vi "tsdiag_can_transfer_data.vi"(6 "AReqCase":i32, 7 "ADataSize":i32, 8 "error in (no error)":errorcluster, 9 "ASourceData":u8[](array[numeric]), 10 "ADiagModuleIndex":i32, 11 "路径输入":path) -> (0 "error out":errorcluster, 1 "Succes？":bool, 2 "return":i32, 3 "路径输出":path)   [LabVIEW 2014]
doc: "36服务，请求传输数据。"
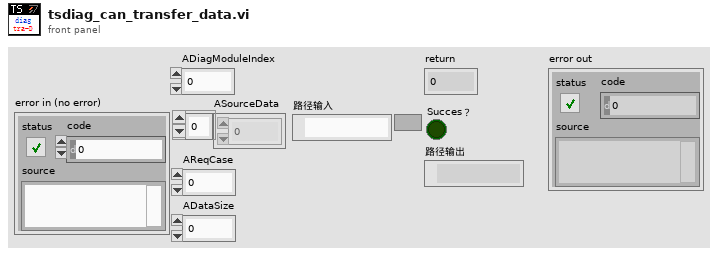
[diagram p1: front panel]
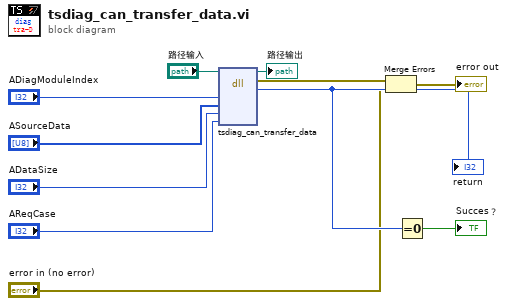
[diagram p0: block diagram]
diagram:
  n1 = dll-call lib="D:/Program Files (x86)/TOSUN/TSMaster/bin/TSMaster.dll" fn="tsdiag_can_transfer_data"(path in="路径输入", "ADiagModuleIndex"="ADiagModuleIndex", "ASourceData"="ASourceData", "ADataSize"="ADataSize", "AReqCase"="AReqCase") -> (path out=→"路径输出":path, error out=w11:errorcluster, "ACode"=w8:i32)  [unwired: 6 in]
  "return" <- w8
  n2 = Merge Errors(w11, "error in (no error)") -> (→"error out":errorcluster)
  n3 = Equal To 0?(x=w8) -> (x = 0?=→"Succes？":bool)
